vi "RedirectMicronPath.vi"(8 "Error In":errorcluster, 10 "Allow Redirect?":bool=TRUE, 11 "Micron Path In":path) -> (0 "Error Out":errorcluster, 2 "Extension":string, 3 "Micron Path Out":path)   [LabVIEW 2019, in "MicronClient.lvclass"]
uses:
  MicronClient.lvclass
  Typedefs/MicronINISection.ctl
  Typedefs/MicronModeINISection.ctl
  <vilib>/Utility/config.llb/NI_LVConfig.lvlib
  <vilib>/SLL Toolkit/SLL File IO/SLL File IO.lvlib
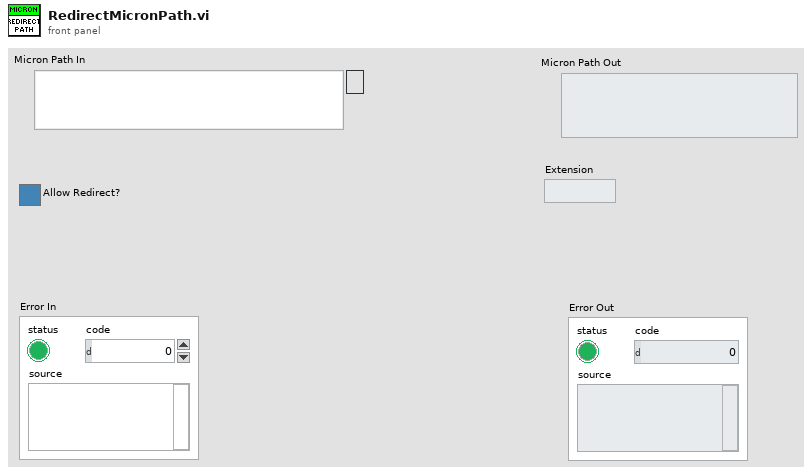
[diagram p1: front panel]
types:
  T1 = typedef "MicronClient.lvclass/MicronModeINISection.ctl" = cluster{"Redirect":string}
  T2 = typedef "MicronClient.lvclass/MicronINISection.ctl" = cluster{"Mode":string}
  T3 = typedef "NI_LVConfig.lvlib/Config Data RefNum.ctl" = refnum<k1>
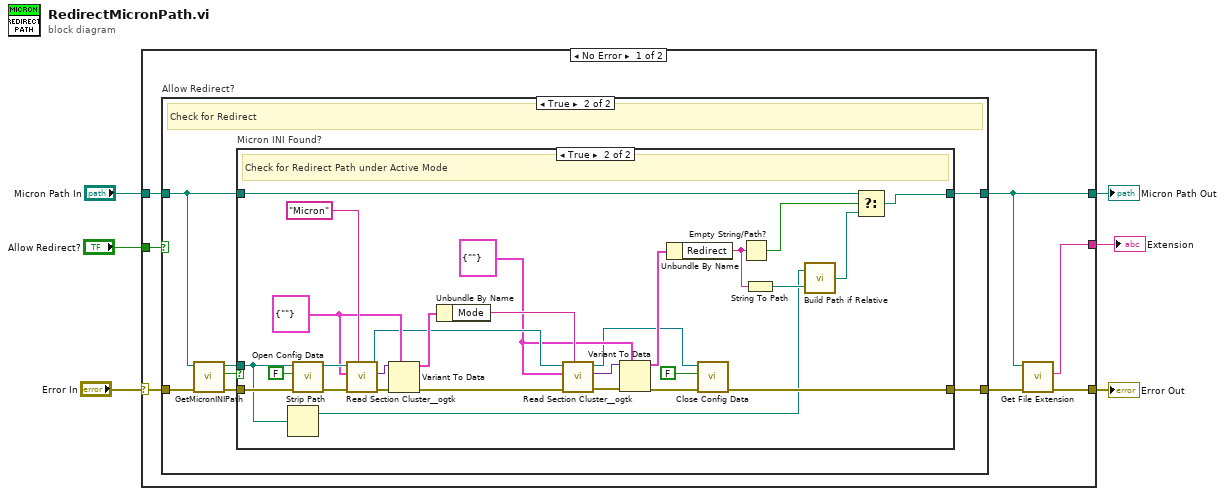
[diagram p0: block diagram]
diagram:
  n1 = case shown="No Error" "Error In" {
    selector: "Error In" -> [w13 w53]
    tunnel: "Micron Path In" -> [w12 w54]
    tunnel: [w8 w53] -> w4
    tunnel: [w10 w54] -> w3
    tunnel: [w9 _] -> w2
    tunnel: "Allow Redirect?" -> [w7 _]
    frame No Error {
      n2 = case "Allow Redirect?" shown="True" w7 {
        tunnel: w13 -> [w14 w22]
        tunnel: w12 -> [w15 w20]
        tunnel: [w14 w17] -> w11
        tunnel: [w15 w16] -> w10
        frame False {
          # "Don't Allow Redirect"
        }
        frame True {
          # "Check for Redirect"
          n3 = call "GetMicronINIPath.vi"("Error In"=w22, "Micron Path In"=w20) -> ("Error Out"=w21:errorcluster, "Present?"=w18:bool, "Micron INI Path Out"=w19:path)  [unwired: 7 in]
          n4 = case "Micron INI Found?" shown="True" w18 {
            tunnel: w21 -> [w23 w52]
            tunnel: w19 -> [_ w27]
            tunnel: w20 -> [w24 w35]
            tunnel: [w24 w30] -> w16
            tunnel: [w23 w29] -> w17
            frame False {
            }
            frame True {
              w38 = T1 {"Redirect"=""} ("Micron Mode")
              w45 = T2 {"Mode"=""} ("Micron")
              # "Check for Redirect Path under Active Mode"
              n5 = Strip Path(path=w27) -> (stripped path=w26:path)  [unwired: 1 out]
              n6 = call <vilib>:"Open Config Data.vi"("error in (no error)"=w52, "create file if necessary (T)"=FALSE, "configuration file path"=w27) -> ("error out"=w51:errorcluster, "refnum"=w48:T3)  [unwired: 6 in, 1 out]
              n7 = call <userlib>:"Read Section Cluster__ogtk.vi"("section (optional)"="Micron", "error in (no error)"=w51, "Section Formatted Cluster Type"=w45, "refnum"=w48) -> ("error out"=w49:errorcluster, "Section Formatted Cluster"=w46:variant, "dup refnum"=w42:T3)  [unwired: 3 in, 2 out]
              n8 = Variant To Data(error in=w49, type=w45, Variant=w46) -> (data=w44:T2, error out=w43:errorcluster)
              n9 = Unbundle By Name(w44) -> ("Mode"=w41:string)
              n10 = call <userlib>:"Read Section Cluster__ogtk.vi"("section (optional)"=w41, "error in (no error)"=w43, "Section Formatted Cluster Type"=w38, "refnum"=w42) -> ("error out"=w40:errorcluster, "Section Formatted Cluster"=w39:variant, "dup refnum"=w32:T3)  [unwired: 3 in, 2 out]
              n11 = Variant To Data(error in=w40, type=w38, Variant=w39) -> (data=w37:T1, error out=w33:errorcluster)
              n12 = Unbundle By Name(w37) -> ("Redirect"=w34:string)
              n13 = call <vilib>:"Close Config Data.vi"("error in (no error)"=w33, "write file if changed (T)"=FALSE, "refnum"=w32) -> ("error out"=w29:errorcluster)  [unwired: 7 in, 1 out]
              n14 = Empty String/Path?(string/path=w34) -> (empty?=w36:bool)
              n15 = String To Path(string=w34) -> (path=w28:path)
              n16 = call <vilib>:"Build Path if Relative.vi"("Relative or Absolute Path"=w28, "Base Path"=w26) -> ("Path Out"=w25:path)
              n17 = Select(t=w35, s=w36, f=w25) -> (s? t:f=w30:path)
            }
          }
        }
      }
      n18 = call <vilib>:"Get File Extension.vi"("error in (no error)"=w11, "file"=w10) -> ("error out"=w8:errorcluster, "lowercase file extension"=w9:string)  [unwired: 5 in, 3 out]
    }
    frame Error {
    }
  }
  "Error Out" <- w4
  "Micron Path Out" <- w3
  "Extension" <- w2
